vi "FGV STOP.vi"(7 "CMD":T1, 8 "error in (no error)":errorcluster, 11 "input":bool) -> (0 "error out":errorcluster, 3 "output":bool)   [LabVIEW 2020]
uses:
  PCT FGV CMD.ctl
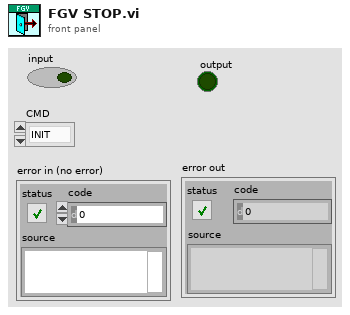
[diagram p1: front panel]
types:
  T1 = typedef "PCT FGV CMD.ctl" = enum16{"INIT", "GET", "SET"}
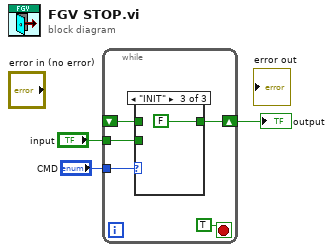
[diagram p0: block diagram]
diagram:
  n1 = while {
    tunnel: "input" -> [w6]
    tunnel: "CMD" -> [w8]
    shift-right: [w5] -> w3
    shift-left: _ -> [w7]
    stop <- TRUE stop-if-true
    n2 = case shown="\"INIT\"" w8 {
      tunnel: w7 -> [_ w10 _]
      tunnel: w6 -> [w9 _ _]
      tunnel: [w9 w10 FALSE ("input")] -> w5
      frame "SET", Default {
      }
      frame "GET" {
      }
      frame "INIT" {
      }
    }
  }
  "output" <- w3
